vi "solar_cfg Read File (Str).vi"(0 "Config Path (*.ini)":path, 1 "Section (\"\" = Use Filename)":string, 2 "Comment":string, 5 "Key":string, 7 "Value in":string, 9 "Add Quotes? (T)":bool=TRUE, 11 "error in (no error)":errorcluster, 13 "Write If Not Found? (T)":bool=TRUE) -> (4 "Config Path out":path, 6 "Value out":string, 10 "Found?":bool, 15 "error out":errorcluster)   [LabVIEW 2018]
doc: "Reads a value associated with a key in a specified section from the configuration file. If the key does not exist and Write If Not Found is True, the VI creates the key in the file. Set a Comment (#...) to add a description after the key's value.\n\n[Section]\nKey = \"Value\" #Comment"
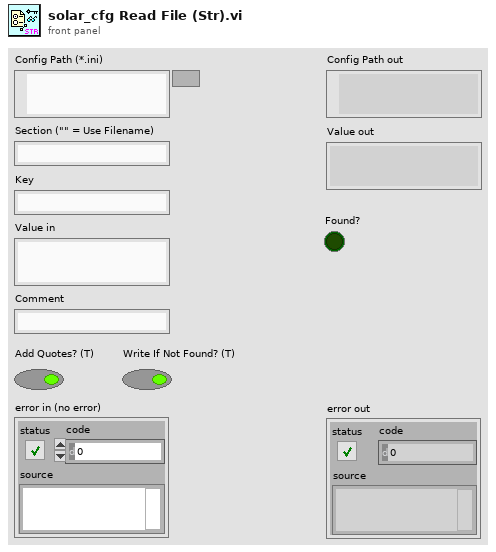
[diagram p1: front panel]
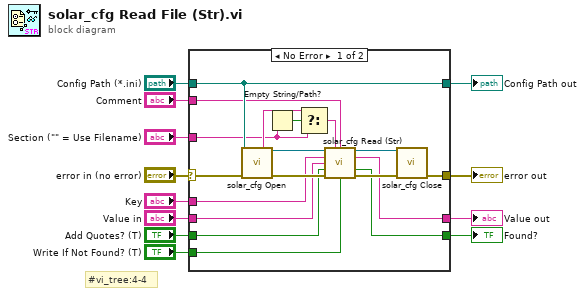
[diagram p0: block diagram]
diagram:
  # "#vi_tree:4-4"
  n1 = case shown="No Error" "error in (no error)" {
    selector: "error in (no error)" -> [w30 w33]
    tunnel: "Config Path (*.ini)" -> [w29 w32]
    tunnel: "Key" -> [w20 _]
    tunnel: [w28 w33] -> w9
    tunnel: "Section (\"\" = Use Filename)" -> [w17 _]
    tunnel: [w14 _] -> w7
    tunnel: [w29 w32] -> w6
    tunnel: "Value in" -> [w21 w31]
    tunnel: [w13 w31] -> w4
    tunnel: "Comment" -> [w15 _]
    tunnel: "Add Quotes? (T)" -> [w23 _]
    tunnel: "Write If Not Found? (T)" -> [w22 _]
    frame No Error {
      n2 = call "solar_cfg Open.vi"("Config Path (*.ini)"=w29, "error in (no error)"=w30) -> ("Filename"=w18:string, "Config Refnum"=w26:refnum<data-value>, "error out"=w27:errorcluster)  [unwired: 10 in, 1 out]
      n3 = Empty String/Path?(string/path=w17) -> (empty?=w19:bool)
      n4 = Select(t=w18, s=w19, f=w17) -> (s? t:f=w16:string)
      n5 = call "solar_cfg Read (Str).vi"("Config Refnum"=w26, "Section"=w16, "Comment"=w15, "Key"=w20, "Value in"=w21, "Add Quotes? (T)"=w23, "error in (no error)"=w27, "Write If Not Found? (T)"=w22) -> ("dup Config Refnum"=w25:refnum<data-value>, "Value out (quotes removed)"=w13:string, "Found?"=w14:bool, "error out"=w24:errorcluster)  [unwired: 4 in]
      n6 = call "solar_cfg Close.vi"("Config Refnum"=w25, "error in (no error)"=w24) -> ("error out"=w28:errorcluster)  [unwired: 12 in, 1 out]
    }
    frame Error {
    }
  }
  "error out" <- w9
  "Config Path out" <- w6
  "Value out" <- w4
  "Found?" <- w7
